vi "PXITrigReserve-Unreserve.vi"(8 "error in":errorcluster, 10 "Mode":enum16{"Reserve", "Unreserve"}(ring)=enum."Unreserve", 11 "FPGA VI Reference In":T1) -> (0 "error out":errorcluster, 3 "FPGA VI Reference Out":T1)   [LabVIEW 2020]
uses:
  Controls/FPGA VI Reference.ctl
  <vilib>/LabVIEW Targets/FPGA/RIO/nirio_PxiTriggers.ctl
  <vilib>/LabVIEW Targets/FPGA/RIO/nirioReserveTrigger.vi
  <vilib>/LabVIEW Targets/FPGA/RIO/nirioUnreserveTrigger.vi
  <vilib>/rvi/interface/nirviMethod/nirviMethod.xnode
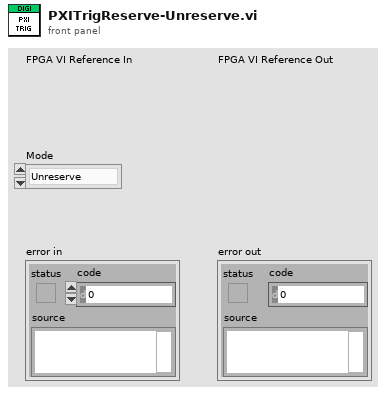
[diagram p1: front panel]
types:
  T1 = typedef "FPGA VI Reference.ctl" = refnum<k20>
  T2 = typedef "nirio_PxiTriggers.ctl" = u16
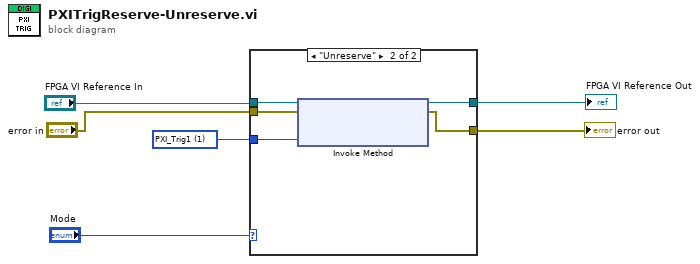
[diagram p0: block diagram]
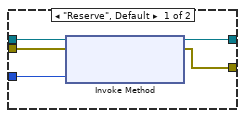
[diagram p2: hidden frame]
diagram:
  w6 = T2 1 items=["PXI_Trig0", "PXI_Trig1", "PXI_Trig2", "PXI_Trig3", "PXI_Trig4", "PXI_Trig5", "PXI_Trig6", "PXI_Trig7"] ("Trigger")
  n1 = case shown="\"Unreserve\"" "Mode" {
    tunnel: w6 -> [w11 w12]
    tunnel: "FPGA VI Reference In" -> [w10 w16]
    tunnel: "error in" -> [w9 w13]
    tunnel: [w8 w15] -> w4
    tunnel: [w7 w14] -> w1
    frame "Reserve", Default {
      n2 = xnode "Invoke Method"("FPGA VI Reference In"=w10, "error in"=w9, "Trigger"=w11) -> ("FPGA VI Reference Out"=w7:T1, "error out"=w8:errorcluster)
    }
    frame "Unreserve" {
      n3 = xnode "Invoke Method"("FPGA VI Reference In"=w16, "error in"=w13, "Trigger"=w12) -> ("FPGA VI Reference Out"=w14:T1, "error out"=w15:errorcluster)
    }
  }
  "error out" <- w4
  "FPGA VI Reference Out" <- w1
